vi "local.Initialize (No Resource).vi"(11 "error in (no error)":errorcluster) -> (4 "SLSC Local out":refnum<class "SLSC Interface.lvclass">, 15 "error out":errorcluster)   [LabVIEW 2016, in "SLSC Interfaces.lvlib" / "SLSC Interface.lvclass"]
uses:
  SLSC Interface Class/SLSC Interface.lvclass
  <vilib>/SLSC/SLSC.lvlib
  <vilib>/SLSC/Initialize Session without Resources.vi
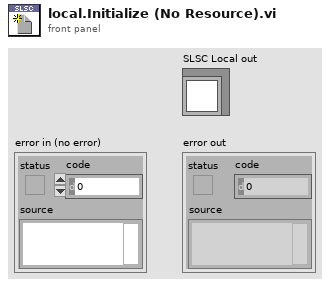
[diagram p1: front panel]
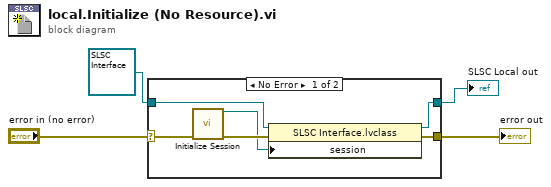
[diagram p0: block diagram]
diagram:
  n1 = case shown="No Error" "error in (no error)" {
    selector: "error in (no error)" -> [w10 w12]
    tunnel: [w6 w12] -> w3
    tunnel: [w8 w11] -> w2
    tunnel: refnum<class "SLSC Interface.lvclass"> refnum ("SLSC Interfaces.lvlib:SLSC Interface.lvclass") -> [w9 w11]
    frame No Error {
      n2 = call-poly <vilib>:"Initialize Session.vi"("error in (no error)"=w10) -> ("session out"=w5:refnum<k21>, "error out"=w7:errorcluster)  [unwired: 13 in]
      n3 = property class="SLSC Interface.lvclass"(reference=w9, error in=w7, "session"=w5) -> (reference out=w8:refnum<class "SLSC Interface.lvclass">, error out=w6:errorcluster)
    }
    frame Error {
    }
  }
  "error out" <- w3
  "SLSC Local out" <- w2
